vi "RearrangeNodes.vi"(0 "reference in":refnum<class "Graph.lvclass">, 5 "error in (no error)":errorcluster) -> (14 "reference out":refnum<class "Graph.lvclass">, 19 "error out":errorcluster)   [LabVIEW 2020, in "Graph.lvclass"]
uses:
  <resource>/Framework/Providers/Open_GDS/UML/Graph_class/Graph.lvclass
  <resource>/Framework/Providers/Open_GDS/UML/AbstractNode_class/AbstractNode.lvclass
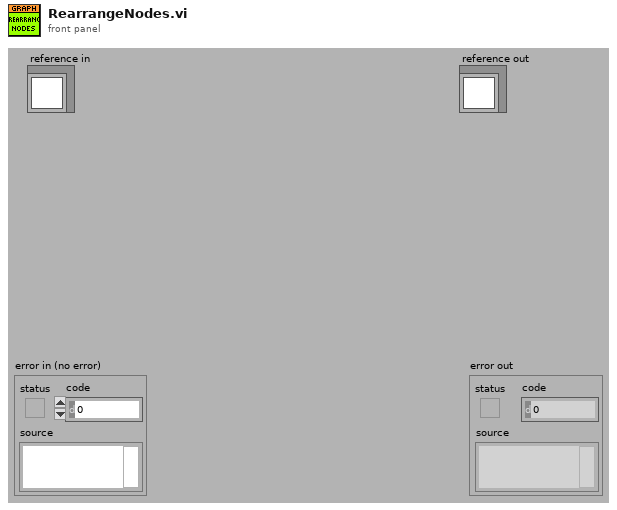
[diagram p1: front panel]
types:
  T1 = typedef "Graph.lvclass/ObjectAttributes.ctl" = cluster{"nodes":refnum<class "AbstractNode.lvclass">[], "edges":refnum<class "AbstractEdge.lvclass">[], "nodesToBeRemoved":refnum<class "AbstractNode.lvclass">[], "edgesToBeRemoved":refnum<class "AbstractEdge.lvclass">[], "needsLayout":bool, "LayoutNodes":refnum<class "AbstractNode.lvclass">[]}
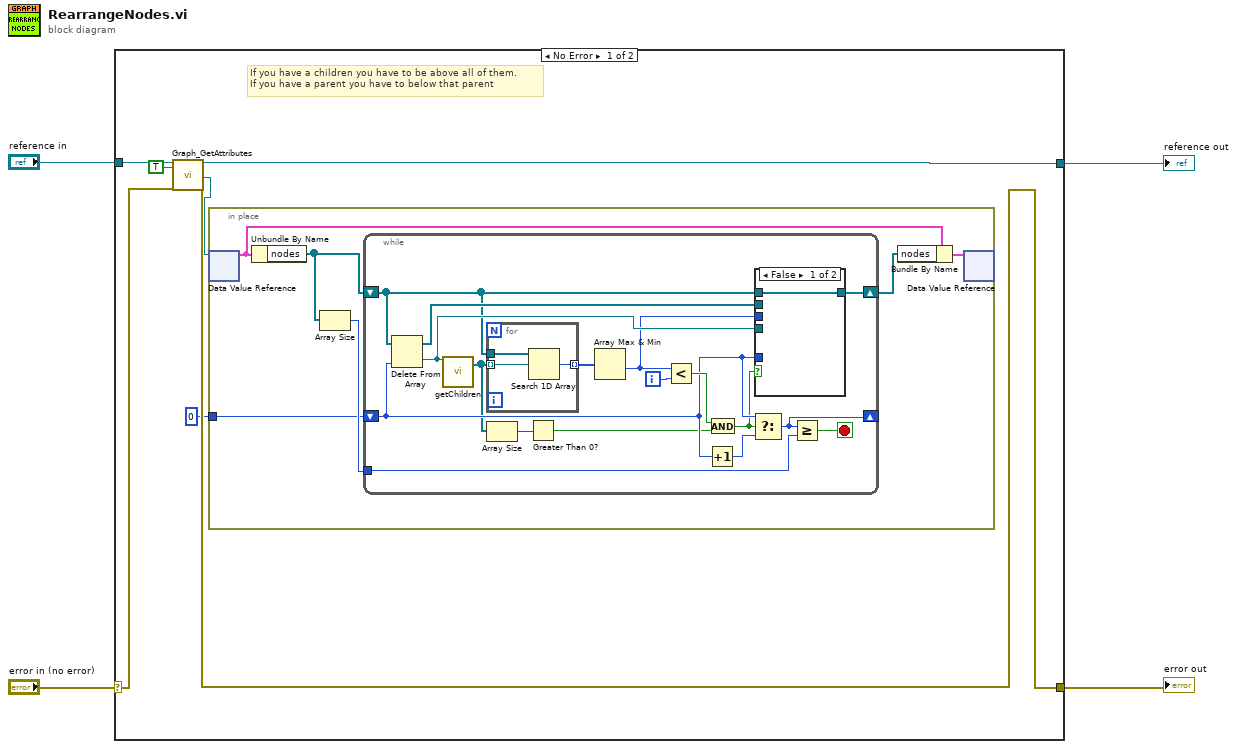
[diagram p0: block diagram]
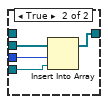
[diagram p2: hidden frame]
diagram:
  n1 = case shown="No Error" "error in (no error)" {
    selector: "error in (no error)" -> [w9 w44]
    tunnel: [w11 w44] -> w3
    tunnel: [w8 w43] -> w1
    tunnel: "reference in" -> [w10 w43]
    frame No Error {
      # "If you have a children you have to be above all of them.\nIf you have a parent you have to below that parent"
      n2 = call <resource>:"Graph_GetAttributes.vi"("reference in"=w10, "OnlyGetDvrReference(False)"=TRUE, "error in (no error)"=w9) -> ("reference out"=w8:refnum<class "Graph.lvclass">, "DataRef"=w6:refnum<data-value>, "error out"=w11:errorcluster)  [unwired: 13 in, 1 out]
      n3 = in-place {
        in-place-border: 0 -> [w12]
        n4 = in-place-dvr #1(w6) -> (w17:T1)  [unwired: 1 out]
        n5 = Unbundle By Name(w17) -> ("nodes"=w16:refnum<class "AbstractNode.lvclass">[])
        n6 = Array Size(array=w16) -> (size(s)=w13:i32)
        n7 = while {
          shift-right: [w25] -> w15
          shift-left: w16 -> [w19]
          shift-right: [w30] -> _
          shift-left: w12 -> [w27]
          tunnel: w13 -> [w32]
          i -> [w33]
          stop <- w31 stop-if-true
          n8 = Delete From Array(array=w19, index=w27) -> (deleted portion=w24:refnum<class "AbstractNode.lvclass">, array with subset deleted=w26:refnum<class "AbstractNode.lvclass">[])  [unwired: 1 in]
          n9 = call-dynamic "getChildren.vi"("reference"=w24) -> ("children"=w23:refnum<class "AbstractNode.lvclass">[])  [unwired: 15 in, 3 out]
          n10 = for {
            tunnel: w23 -> [w42] mode=indexing
            tunnel: w19 -> [w41]
            tunnel: [w40] -> w34 mode=indexing
            n11 = Search 1D Array(1D array=w41, element=w42) -> (index of element=w40:i32)  [unwired: 1 in]
          }
          n12 = Array Size(array=w23) -> (size(s)=w22:i32)
          n13 = Greater Than 0?(x=w22) -> (x > 0?=w20:bool)
          n14 = Array Max & Min(array=w34) -> (min value=w18:i32)  [unwired: 3 out]
          n15 = Less?(x=w18, y=w33) -> (x < y?=w28:bool)
          n16 = Increment(x=w27) -> (x+1=w29:i32)
          n17 = And(x=w28, y=w20) -> (x .and. y?=w21:bool)
          n18 = Select(t=w27, s=w21, f=w29) -> (s? t:f=w30:i32)
          n19 = case shown="False" w21 {
            tunnel: w27 -> [_ _]
            tunnel: w26 -> [_ w39]
            tunnel: [w35 w38] -> w25
            tunnel: w24 -> [_ w37]
            tunnel: w18 -> [_ w36]
            tunnel: w19 -> [w35 _]
            frame False {
            }
            frame True {
              n20 = Insert Into Array(array=w39, index=w36, new element=w37) -> (w38:refnum<class "AbstractNode.lvclass">[])
            }
          }
          n21 = Greater Or Equal?(x=w30, y=w32) -> (x >= y?=w31:bool)
        }
        n22 = Bundle By Name(cluster=w17, "nodes"=w15) -> (w14:T1)
        n23 = in-place-dvr #1(w14) -> ()  [unwired: 2 out]
      }
    }
    frame Error {
    }
  }
  "error out" <- w3
  "reference out" <- w1
